vi "sensorsLoop.vi"() -> ()   [LabVIEW 2018]
uses:
  <vilib>/Rock Robotics/WPI/ThirdParty/Phoenix-LabVIEW/Motor Controller/Controls/CTRE_Phoenix_MotorControl_StatusFrameEnhanced.ctl
  <vilib>/Platform/TimedLoop/XDataNode/timing_clust.ctl
  <vilib>/Platform/TimedLoop/XDataNode/nitl_modes.ctl
  <vilib>/Platform/TimedLoop/XDataNode/wakeup.ctl
  Drive/driveShifterEnum.ctl
  Drive/MotionProfile/Constants.vi
  <vilib>/Rock Robotics/WPI/ThirdParty/Phoenix-LabVIEW/Motor Controller/Get/CTRE_Phoenix_MotorController_GetSelectedSensorData.vi
  <vilib>/Rock Robotics/WPI/ThirdParty/Phoenix-LabVIEW/Motor Controller/Get/CTRE_Phoenix_MotorController_GetQuadratureData.vi
  <vilib>/Rock Robotics/WPI/ThirdParty/Phoenix-LabVIEW/Pigeon IMU/CTRE_PigeonIMU_GetFusedHeading.vi
  <vilib>/Rock Robotics/WPI/ThirdParty/Phoenix-LabVIEW/Pigeon IMU/CTRE_PigeonIMU_GetBiasedAccelerometer.vi
  <vilib>/Rock Robotics/WPI/ThirdParty/Phoenix-LabVIEW/Pigeon IMU/CTRE_PigeonIMU_GetYPR.vi
  <vilib>/platform/TimedLoop/XDataNode/XDataNode.xnode
  <vilib>/Platform/TimedLoop/XDataNode/XDNodeRunTimeDep.lvlib
  <userlib>/836-Library/System/TDMS_V2/Support/TDMS_DevRef.ctl
  <userlib>/836-Library/System/TDMS_V2/Support/Logging_Settings.ctl
  <userlib>/836-Library/System/TDMS_V2/Support/Group_FIFO_Config.ctl
  <userlib>/836-Library/System/TDMS_V2/Support/Channel_FIFO_Config.ctl
panel:
  out "max 2":dbl
  out "velocity max_min 2":cluster{"min":dbl, "max":dbl, dbl}(graph)
  out "min 2":dbl
  out "Cal Status":T1
  in  "Read Enable":T2={"Cal Status"=TRUE, "Orientation"=TRUE, "Gyro"=FALSE, "Accelerometer"=FALSE, "Quanterion"=FALSE, "Accel Mode"=enum."Linear", "Magnetometer"=FALSE, "Register Mode"=enum."Quaternion"}
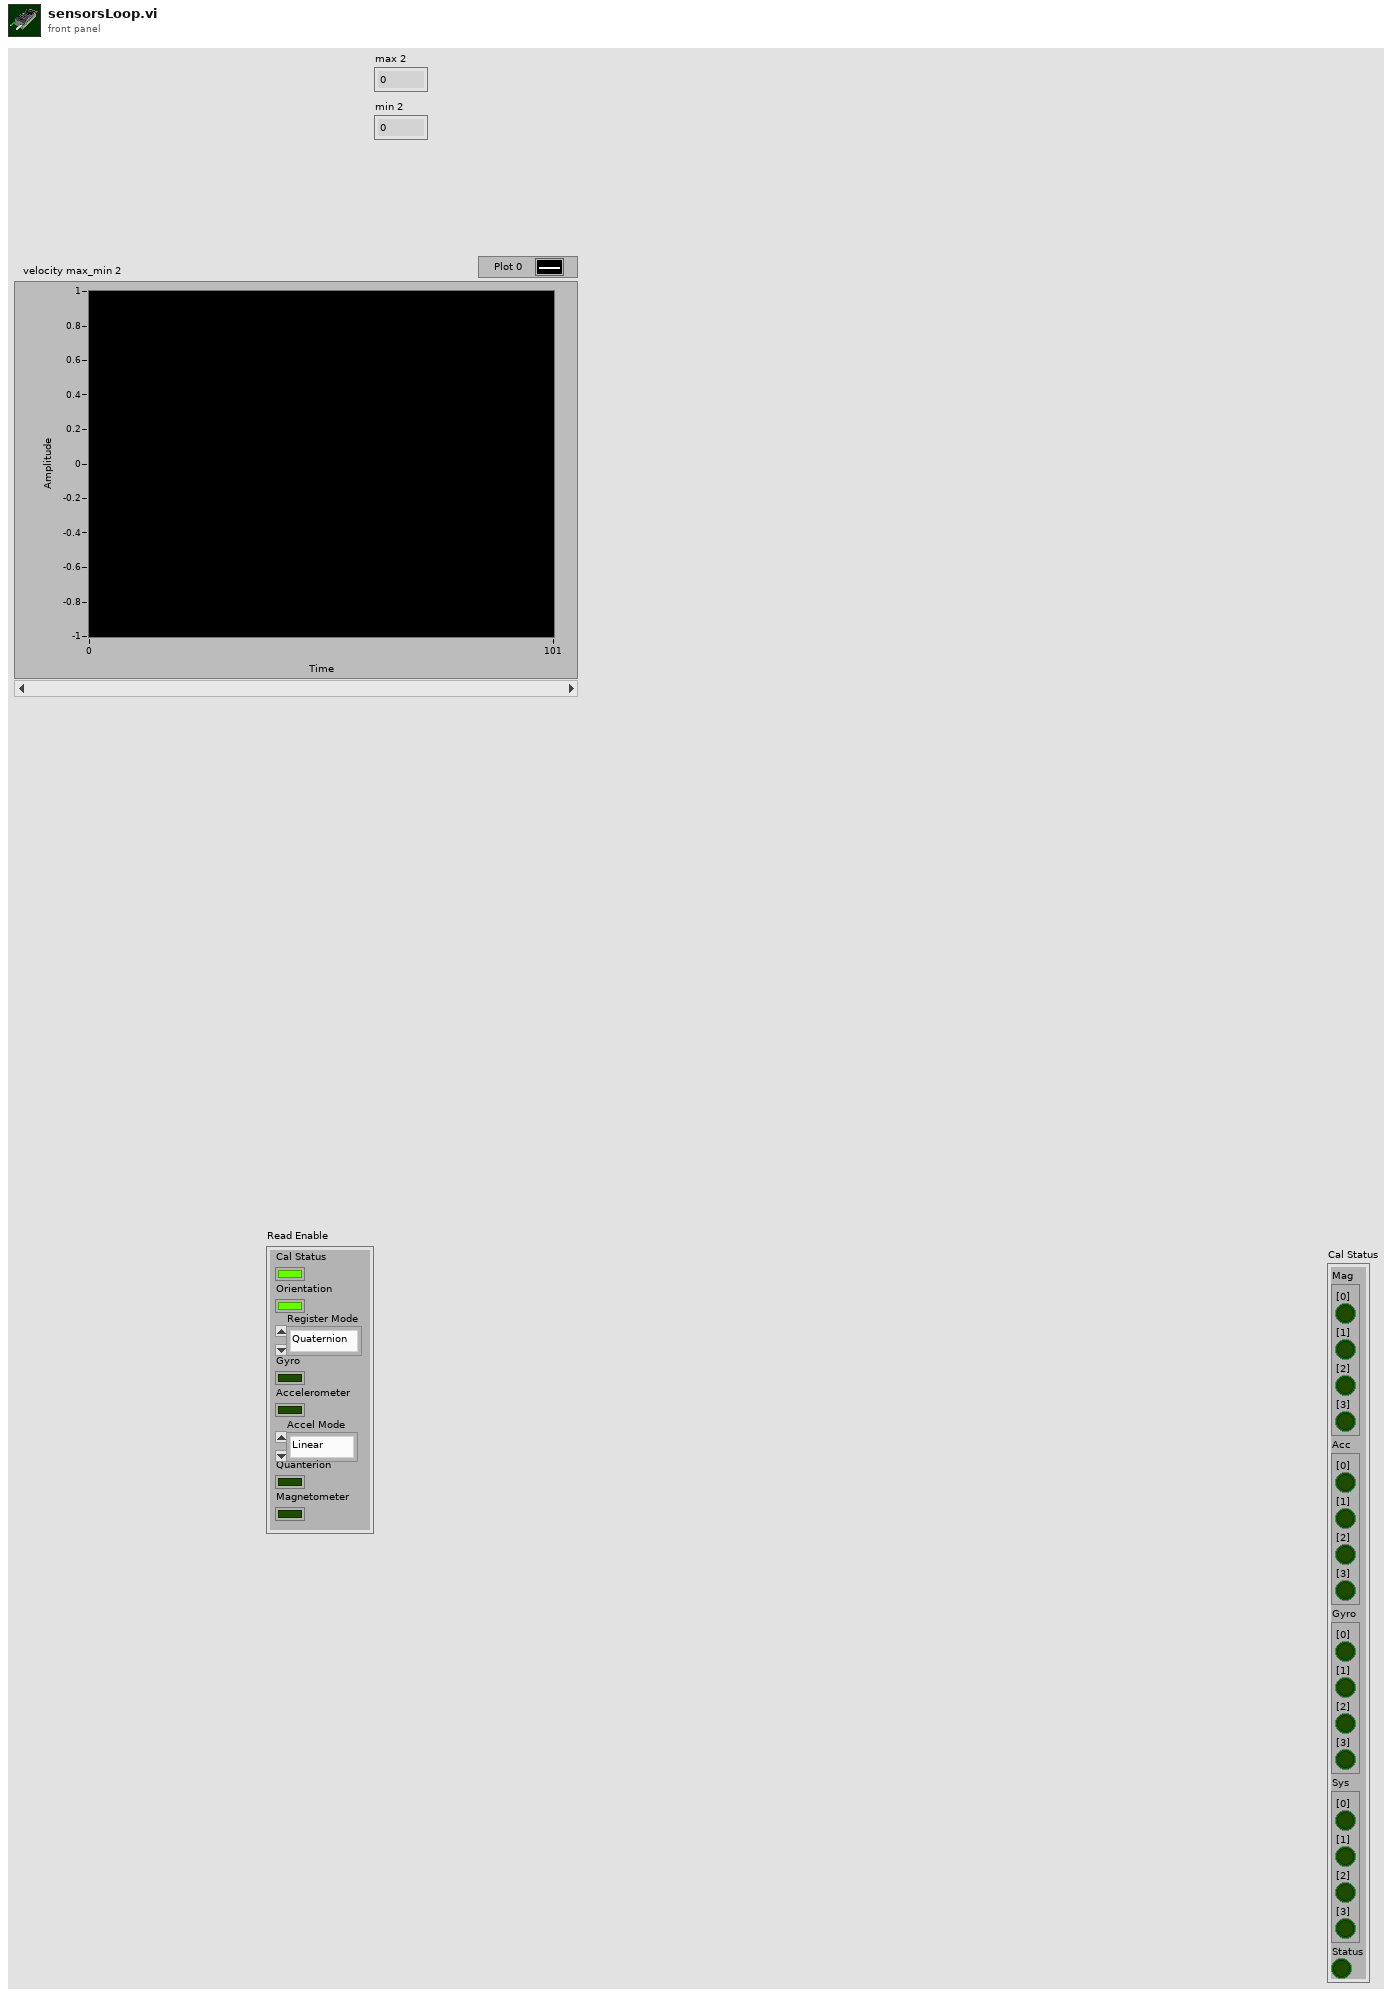
[diagram p1: front panel]
types:
  T1 = cluster{"Mag":cluster{"[0]":bool, "[1]":bool, "[2]":bool, "[3]":bool}, "Acc":cluster{"[0]":bool, "[1]":bool, "[2]":bool, "[3]":bool}, "Gyro":cluster{"[0]":bool, "[1]":bool, "[2]":bool, "[3]":bool}, "Sys":cluster{"[0]":bool, "[1]":bool, "[2]":bool, "[3]":bool}, "Status":bool}
  T2 = cluster{"Cal Status":bool, "Orientation":bool, "Gyro":bool, "Accelerometer":bool, "Quanterion":bool, "Accel Mode":enum8{"Raw Data", "Linear", "Gravity"}, "Magnetometer":bool, "Register Mode":enum8{"Euler", "Quaternion"}}
  T3 = typedef "CTRE_Phoenix_MotorControl_StatusFrameEnhanced.ctl" = u16
  T4 = typedef "WPI_MotorControlDeviceRef.ctl" = cluster{"DeviceStatus":errorcluster, "Type":T5, "PWM":cluster{"PWM Channel":T6, "DeadBand":T7}, "CAN":cluster{"Device Number":u8, "SetOutput VI Ref":variant, "GetOutput VI Ref":variant, "Enable VI Ref":variant, "Disable VI Ref":variant, "Data":variant}, "Invert":bool, "DIO PWM":cluster{"PWM \"Enable\" Channel":T6, "DIOChannel":T8, "PWM Rate":dbl}}
  T5 = typedef "WPI_MotorControlType.ctl" = enum16{"PWM", "CAN", "DIO PWM"}
  T6 = typedef "FPGA_DIOPWMChannel.ctl" = enum8{"PWM 0", "PWM 1", "PWM 2", "PWM 3", "PWM 4", "PWM 5", "PWM 6", "PWM 7", "PWM 8", "PWM 9", "PWM MXP 0", "PWM MXP 1", "PWM MXP 2", "PWM MXP 3", "PWM MXP 4", "PWM MXP 5", "PWM MXP 6", "PWM MXP 7", "PWM MXP 8", "PWM MXP 9", "Invalid"}
  T7 = typedef "WPI_PWMDeadband.ctl" = cluster{"Name":string, "maxPositivePwm":i32, "minPositivePwm":i32, "centerPwm":i32, "maxNegativePwm":i32, "minNegativePwm":i32, "angularRange":u16}
  T8 = typedef "FPGA_DIOChannel.ctl" = enum8{"DIO 0", "DIO 1", "DIO 2", "DIO 3", "DIO 4", "DIO 5", "DIO 6", "DIO 7", "DIO 8", "DIO 9", "DIO MXP 0", "DIO MXP 1", "DIO MXP 2", "DIO MXP 3", "DIO MXP 4", "DIO MXP 5", "DIO MXP 6", "DIO MXP 7", "DIO MXP 8", "DIO MXP 9", "DIO MXP 10", "DIO MXP 11", "DIO MXP 12", "DIO MXP 13", "DIO MXP 14", "DIO MXP 15", "SPI Port CS1", "SPI Port CS2", "SPI Port CS3", "SPI Port MISO", "SPI Port MOSI", "Invalid"}
  T9 = typedef "WPI_AnalogChannelDevRef.ctl" = cluster{"DevStatus":errorcluster, "Analog Channel":T10}
  T10 = typedef "FPGA_AIChannel.ctl" = enum8{"AI 0", "AI 1", "AI 2", "AI 3", "AI MXP 0", "AI MXP 1", "AI MXP 2", "AI MXP 3", "Invalid"}
  T11 = typedef "CTRE_PigeonIMU_DeviceRef.ctl" = cluster{"DeviceStatus":errorcluster, "Device Number":u8, "Type":T12, "Device ID":u32, "Handle":u64, "UsageFrame":u32, "Library Path":path}
  T12 = typedef "CTRE_PigeonIMU_ConnectionType.ctl" = u32
  T13 = typedef "WPI_DigitalInputDevRef.ctl" = cluster{"DevStatus":errorcluster, "DIO Channel":T8}
  T14 = typedef "XDNodeRunTimeDep.lvlib/timing_clust.ctl" = cluster{"Expected End [f-1]":u64, "Actual End [f-1]":u64, "Finished Late? [f-1]":bool, "Expected End [i-1]":u64, "Actual End [i-1]":u64, "Finished Late? [i-1]":bool, "Expected Start [i]":u64, "Actual Start [i]":u64, "Expected Start [f]":u64, "Actual Start [f]":u64, "Source Name":string, "Structure Name":string, "Period":i64, "Deadline":i64, "Offset":i64, "Start":i64, "Priority":i32, "Timeout":i32, "Mode":T15, "Wakeup Reason":T16, "Error":errorcluster, "Source Type":string, "Secondary Source Type":string, "Global End Time":u64, "Global Start Time":u64, "Frame Duration":u64, "Iteration Duration":u64, "Assigned CPU":i32, "I/O Scan Engine Mode":u32}
  T15 = typedef "XDNodeRunTimeDep.lvlib/nitl_modes.ctl" = enum32{"No Change", "Process missed periods, maintain original phase", "Discard missed periods, maintain original phase", "Process missed periods, ignore original phase", "Discard missed periods, ignore original phase"}
  T16 = typedef "XDNodeRunTimeDep.lvlib/wakeup.ctl" = enum32{"Normal", "Aborted", "Asynchronous wakeup", "Timing source error", "Timed loop error", "Timeout"}
  T17 = typedef "ImuDevRef.ctl" = cluster{"I2CDevRef":T18, "Valid Cal File?":bool}
  T18 = typedef "WPI_I2CDevRef.ctl" = cluster{"DevStatus":errorcluster, "Device Address":u8, "Handle":i32, "I2C Bus":T19}
  T19 = typedef "i2c_bus.ctl" = enum16{"I2C On-Board", "I2C MXP", "Invalid"}
  T20 = enum16{"Inches -> Sensor Units", "Sensor Units -> Inches"}
  T21 = typedef "driveShifterEnum.ctl" = enum16{"Low", "High"}
  T22 = cluster{"Heading":dbl, "Valid?":bool, "Fusing?":bool}
  T23 = typedef "TDMS_DevRef.ctl" = cluster{"Name":string, "File Ref":refnum<k34>, "Start Time":timestamp, "Logging Settings":T24, "Group FIFO Config":T25[], "Data To Write":refnum<data-value>, "semaphore":T27, "Ref Time Reset":refnum<k4>}
  T24 = typedef "Logging_Settings.ctl" = cluster{"Data Grab Period":dbl, "File Write Period":dbl, "Max Stored Size":dbl, "Burst Size":dbl}
  T25 = typedef "Group_FIFO_Config.ctl" = cluster{"Group":string, "Channels":T26[], "Channel Names":string[]}
  T26 = typedef "Channel_FIFO_Config.ctl" = cluster{"Channel":string, "FIFO":refnum<k33>}
  T27 = typedef "Semaphore RefNum" = refnum<k1>
  T28 = cluster{"Yaw":dbl, "Roll":dbl, "Pitch":dbl, "Yaw Wind":dbl, "Roll Wind":dbl, "Pitch Wind":dbl}
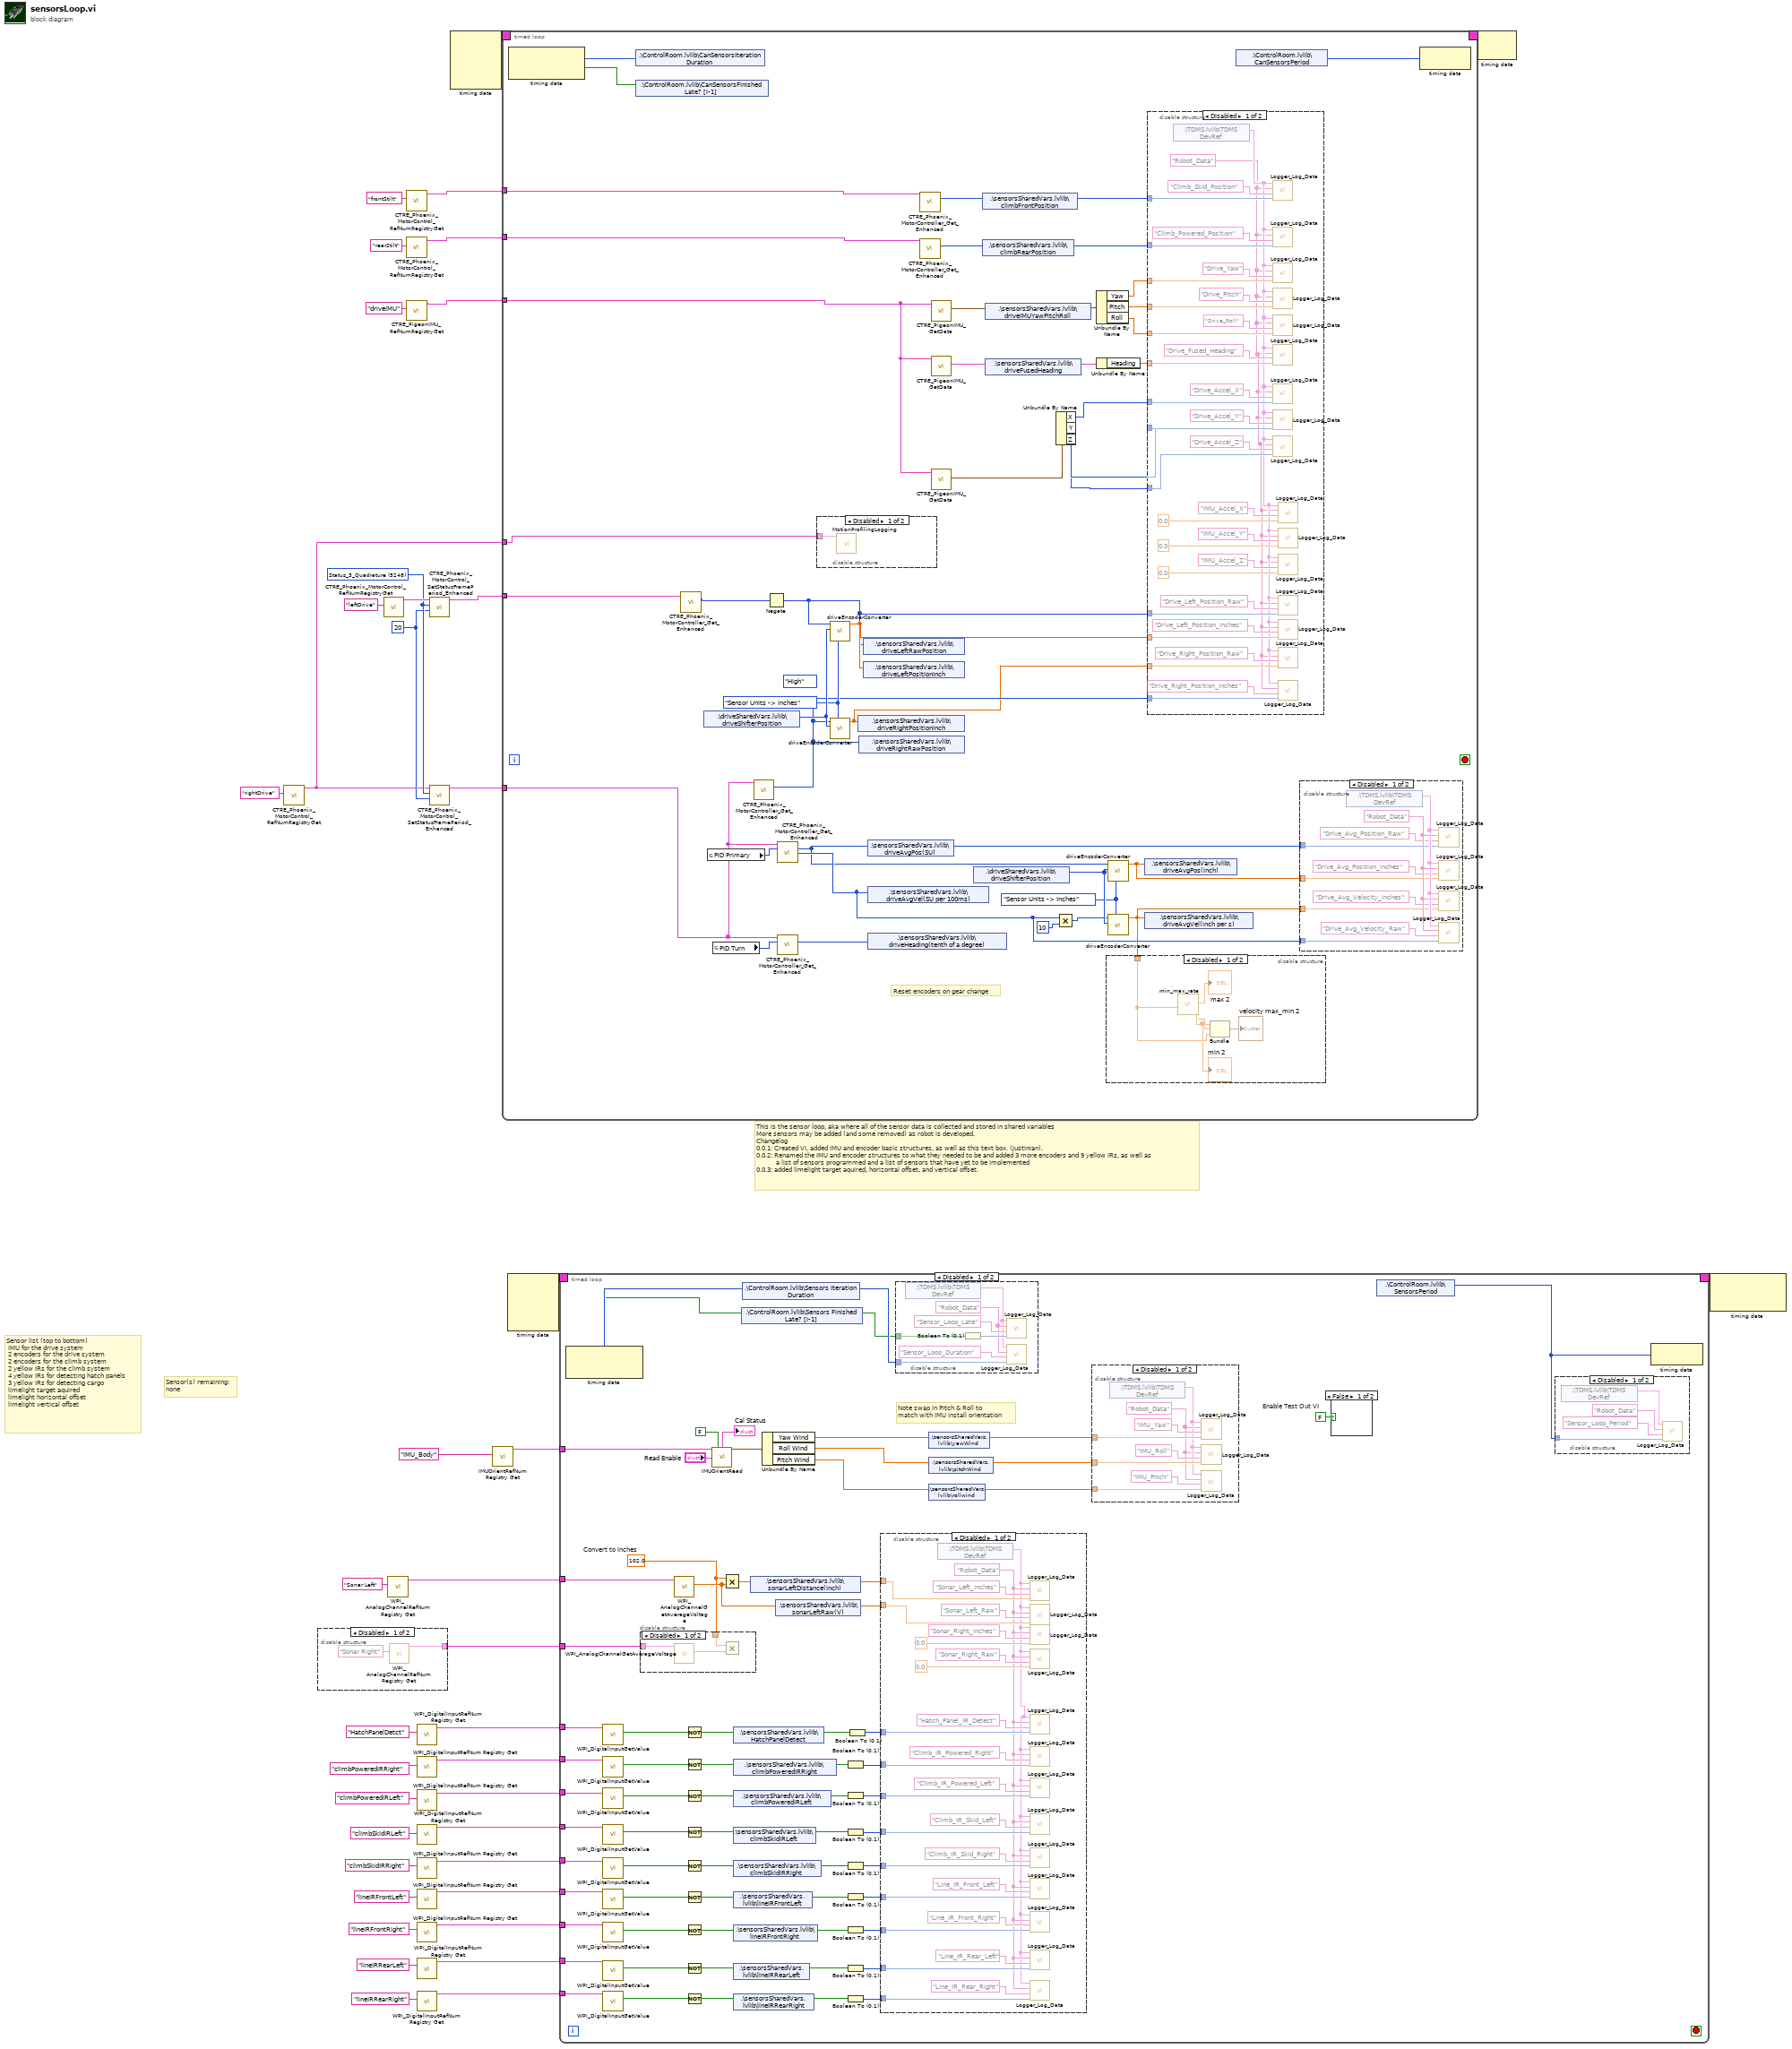
[diagram p0: block diagram]
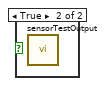
[diagram p12: hidden frame]
diagram:
  w4 = 20 ("periodMs")
  w5 = T3 5248 items=["Status_1_General"=5120, "Status_2_Feedback0"=5184, "Status_3_Quadrature"=5248, "Status_4_AinTempVbat"=5312, "Status_6_Misc"=5440, "Status_7_CommStatus"=5504, "Status_8_PulseWidth"=5568, "Status_9_MotProfBuffer"=5632, "Status_10_MotionMagic"=5696, "Status_11_UartGadgeteer"=5760, "Status_12_Feedback1"=5824, "Status_13_Base_PIDF0"=5888, "Status_14_Turn_PIDF1"=5952, "Status_15_FirmwareApiStatus"=6016] ("Status Frame")
  # "Sensor(s) remaining:\nnone"
  # "Sensor list (top to bottom)\n IMU for the drive system\n 2 encoders for the drive system\n 2 encoders for the climb system\n 2 yellow IRs for the climb system\n 4 yellow IRs for detecting hatch panels\n 3 yellow IRs for detecting cargo\n limelight target aquired\n limelight horizontal offset\n limelight vertical offset"
  # "This is the sensor loop, aka where all of the sensor data is collected and stored in shared variables\nMore sensors may be added (and some removed) as robot is developed.\nChangelog\n0.0.1: Created VI, added IMU and encoder basic structures, as well as this text box. (Justinian).\n0.0.2: Renamed the IMU and encoder structures to what they needed to be and added 3 more encoders and 9 yellow IRs, as well as\n           a list of sensors programmed and a list of sensors that have yet to be implemented\n0.0.3: added limelight target aquired, horizontal offset, and vertical offset."
  n1 = call <vilib>:"CTRE_Phoenix_MotorControl_RefNumRegistryGet.vi"("refnum name"="rightDrive") -> ("PhoenixMotorControlDevRef"=w2:T4)  [unwired: 9 in, 1 out]
  n2 = disable-structure shown="Disabled" {
    disable-tunnel: [w43 _] -> w19
    frame Disabled {
      n3 = call <vilib>:"WPI_AnalogChannelRefNum Registry Get.vi"("refnum name"="Sonar Right") -> ("AIDeviceRef"=w43:T9)  [unwired: 9 in, 1 out]
    }
    frame Enabled {
    }
  }
  n4 = call <vilib>:"CTRE_Phoenix_MotorControl_RefNumRegistryGet.vi"("refnum name"="leftDrive") -> ("PhoenixMotorControlDevRef"=w6:T4)  [unwired: 9 in, 1 out]
  n5 = call <vilib>:"WPI_AnalogChannelRefNum Registry Get.vi"("refnum name"="Sonar Left") -> ("AIDeviceRef"=w20:T9)  [unwired: 9 in, 1 out]
  n6 = call <vilib>:"CTRE_Phoenix_MotorControl_RefNumRegistryGet.vi"("refnum name"="frontStilt") -> ("PhoenixMotorControlDevRef"=w11:T4)  [unwired: 9 in, 1 out]
  n7 = call <vilib>:"CTRE_Phoenix_MotorControl_RefNumRegistryGet.vi"("refnum name"="rearStilt") -> ("PhoenixMotorControlDevRef"=w10:T4)  [unwired: 9 in, 1 out]
  n8 = call <vilib>:"CTRE_PigeonIMU_RefNumRegistryGet.vi"("refnum name"="driveIMU") -> ("PigeonIMUDevRef"=w9:T11)  [unwired: 9 in, 1 out]
  n9 = call <vilib>:"WPI_DigitalInputRefNum Registry Get.vi"("refnum name"="HatchPanelDetct") -> ("DigitalInputDevRef"=w17:T13)  [unwired: 9 in, 1 out]
  n10 = call <vilib>:"WPI_DigitalInputRefNum Registry Get.vi"("refnum name"="climbPoweredIRRight") -> ("DigitalInputDevRef"=w30:T13)  [unwired: 9 in, 1 out]
  n11 = call <vilib>:"WPI_DigitalInputRefNum Registry Get.vi"("refnum name"="climbPoweredIRLeft") -> ("DigitalInputDevRef"=w29:T13)  [unwired: 9 in, 1 out]
  n12 = call <vilib>:"WPI_DigitalInputRefNum Registry Get.vi"("refnum name"="climbSkidIRLeft") -> ("DigitalInputDevRef"=w28:T13)  [unwired: 9 in, 1 out]
  n13 = call <vilib>:"WPI_DigitalInputRefNum Registry Get.vi"("refnum name"="climbSkidIRRight") -> ("DigitalInputDevRef"=w27:T13)  [unwired: 9 in, 1 out]
  n14 = call <vilib>:"WPI_DigitalInputRefNum Registry Get.vi"("refnum name"="lineIRFrontLeft") -> ("DigitalInputDevRef"=w26:T13)  [unwired: 9 in, 1 out]
  n15 = call <vilib>:"WPI_DigitalInputRefNum Registry Get.vi"("refnum name"="lineIRFrontRight") -> ("DigitalInputDevRef"=w25:T13)  [unwired: 9 in, 1 out]
  n16 = call <vilib>:"WPI_DigitalInputRefNum Registry Get.vi"("refnum name"="lineIRRearLeft") -> ("DigitalInputDevRef"=w24:T13)  [unwired: 9 in, 1 out]
  n17 = call <vilib>:"WPI_DigitalInputRefNum Registry Get.vi"("refnum name"="lineIRRearRight") -> ("DigitalInputDevRef"=w23:T13)  [unwired: 9 in, 1 out]
  n18 = call <vilib>:"CTRE_Phoenix_MotorControl_SetStatusFramePeriod_Enhanced.vi"("periodMs"=w4, "Status Frame"=w5, "PhoenixMotorControlDevRef"=w6) -> ("PhoenixMotorControlDevRef"=w3:T4)  [unwired: 7 in, 1 out]
  n19 = call <vilib>:"CTRE_Phoenix_MotorControl_SetStatusFramePeriod_Enhanced.vi"("periodMs"=w4, "Status Frame"=w5, "PhoenixMotorControlDevRef"=w2) -> ("PhoenixMotorControlDevRef"=w1:T4)  [unwired: 7 in, 1 out]
  n20 = node-c288() -> (w16:T14)  [unwired: 4 in]
  n21 = call <userlib>:"IMUOrientRefNum Registry Get.vi"("refnum name"="IMU_Body") -> ("IMUDevRef out"=w39:T17)  [unwired: 9 in, 1 out]
  n22 = timed-loop {
    timing: w16 -> [_]
    timing-out: [_] -> w15
    tunnel: w11 -> [w70]
    tunnel: w10 -> [w69]
    tunnel: w9 -> [w68]
    tunnel: w3 -> [w54]
    tunnel: w2 -> [w56]
    tunnel: w1 -> [w55]
    stop <- _ stop-if-true
    w47 = T20."Sensor Units -> Inches" ("Conversion Direction")
    (unwired) enum16{"High", "Low"}."High" ("Gear Setting")
    w66 = T20."Sensor Units -> Inches" ("Conversion Direction")
    # "Reset encoders on gear change"
    n23 = node-c288() -> (w53:i64, w52:bool)  [unwired: 1 in]
    n24 = shared-variable ".\\ControlRoom.lvlib\\CanSensorsIteration Duration"(w53) -> ()  [unwired: 1 in, 1 out]
    n25 = shared-variable ".\\ControlRoom.lvlib\\CanSensorsFinished Late? [i-1]"(w52) -> ()  [unwired: 1 in, 1 out]
    n26 = call-poly <vilib>:"CTRE_Phoenix_MotorController_Get_Enhanced.vi"("PhoenixMotorControlDevRef"=w54) -> ("Quadrature Position"=w58:i32)  [unwired: 11 in, 3 out]
    n27 = shared-variable ".\\driveSharedVars.lvlib\\driveShifterPosition"() -> (w67:T21)  [unwired: 1 in, 1 out]
    n28 = global read "Constants.vi" "PID Primary"() -> (w44:i32)
    n29 = global read "Constants.vi" "PID Turn"() -> (w45:i32)
    n30 = call-poly <vilib>:"CTRE_Phoenix_MotorController_Get_Enhanced.vi"("PhoenixMotorControlDevRef"=w55) -> ("Quadrature Position"=w62:i32)  [unwired: 11 in, 3 out]
    n31 = Negate(x=w58) -> (-x=w59:i32)
    n32 = call-poly <vilib>:"CTRE_Phoenix_MotorController_Get_Enhanced.vi"("PhoenixMotorControlDevRef"=w55, "pidLoopIdx"=w44) -> ("Position (Raw Sensor Units)"=w63:i32, "Velocity (Raw Sensor Units per 100 ms)"=w65:i32)  [unwired: 10 in, 2 out]
    n33 = call-poly <vilib>:"CTRE_Phoenix_MotorController_Get_Enhanced.vi"("PhoenixMotorControlDevRef"=w55, "pidLoopIdx"=w45) -> ("Position (Raw Sensor Units)"=w46:i32)  [unwired: 10 in, 3 out]
    n34 = disable-structure shown="Disabled" {
      disable-tunnel: w56 -> [w127 _]
      frame Disabled {
        n35 = call "MotionProfilingLogging.vi"("Main Talon"=w127) -> ()  [unwired: 11 in]
      }
      frame Enabled {
      }
    }
    n36 = call "driveEncoderConverter.vi"("Conversion Direction"=w66, "Gear Setting"=w67, "Input"=w59) -> ("Output"=w60:dbl)  [unwired: 8 in]
    n37 = call "driveEncoderConverter.vi"("Conversion Direction"=w66, "Gear Setting"=w67, "Input"=w62) -> ("Output"=w61:dbl)  [unwired: 8 in]
    n38 = shared-variable ".\\sensorsSharedVars.lvlib\\driveRightPositionInch"(w61) -> ()  [unwired: 1 in, 1 out]
    n39 = shared-variable ".\\sensorsSharedVars.lvlib\\driveRightRawPosition"(w62) -> ()  [unwired: 1 in, 1 out]
    n40 = shared-variable ".\\sensorsSharedVars.lvlib\\driveLeftPositionInch"(w60) -> ()  [unwired: 1 in, 1 out]
    n41 = shared-variable ".\\sensorsSharedVars.lvlib\\driveLeftRawPosition"(w59) -> ()  [unwired: 1 in, 1 out]
    n42 = shared-variable ".\\sensorsSharedVars.lvlib\\driveAvgPos(SU)"(w63) -> ()  [unwired: 1 in, 1 out]
    n43 = shared-variable ".\\sensorsSharedVars.lvlib\\driveAvgVel(SU per 100ms)"(w65) -> ()  [unwired: 1 in, 1 out]
    n44 = shared-variable ".\\sensorsSharedVars.lvlib\\driveHeading(tenth of a degree)"(w46) -> ()  [unwired: 1 in, 1 out]
    n45 = call-poly <vilib>:"CTRE_Phoenix_MotorController_Get_Enhanced.vi"("PhoenixMotorControlDevRef"=w70) -> ("Position (Raw Sensor Units)"=w82:i32)  [unwired: 11 in, 3 out]
    n46 = call-poly <vilib>:"CTRE_Phoenix_MotorController_Get_Enhanced.vi"("PhoenixMotorControlDevRef"=w69) -> ("Position (Raw Sensor Units)"=w81:i32)  [unwired: 11 in, 3 out]
    n47 = call-poly <vilib>:"CTRE_PigeonIMU_GetData.vi"("PigeonIMUDevRef"=w68) -> ("Yaw Pitch Roll"=w72:cluster{"Yaw":dbl, "Pitch":dbl, "Roll":dbl})  [unwired: 8 in, 2 out]
    n48 = call-poly <vilib>:"CTRE_PigeonIMU_GetData.vi"("PigeonIMUDevRef"=w68) -> ("Fused Heading"=w71:T22)  [unwired: 8 in, 2 out]
    n49 = call-poly <vilib>:"CTRE_PigeonIMU_GetData.vi"("PigeonIMUDevRef"=w68) -> ("Biased Accelerometer"=w76:cluster{"X":i16, "Y":i16, "Z":i16, "Norm":i16})  [unwired: 8 in, 2 out]
    n50 = shared-variable ".\\driveSharedVars.lvlib\\driveShifterPosition"() -> (w50:T21)  [unwired: 1 in, 1 out]
    n51 = shared-variable ".\\sensorsSharedVars.lvlib\\climbFrontPosition"(w82) -> ()  [unwired: 1 in, 1 out]
    n52 = shared-variable ".\\sensorsSharedVars.lvlib\\climbRearPosition"(w81) -> ()  [unwired: 1 in, 1 out]
    n53 = shared-variable ".\\sensorsSharedVars.lvlib\\driveIMUYawPitchRoll"(w72) -> ()  [unwired: 1 in, 1 out]
    n54 = shared-variable ".\\sensorsSharedVars.lvlib\\driveFusedHeading"(w71) -> ()  [unwired: 1 in, 1 out]
    n55 = Multiply(x=w65, y=10) -> (x*y=w48:i32)
    n56 = Unbundle By Name(w76) -> ("X"=w74:i16, "Y"=w75:i16, "Z"=w73:i16)
    n57 = Unbundle By Name(w72) -> ("Yaw"=w80:dbl, "Pitch"=w79:dbl, "Roll"=w78:dbl)
    n58 = Unbundle By Name(w71) -> ("Heading"=w77:dbl)
    n59 = call "driveEncoderConverter.vi"("Conversion Direction"=w47, "Gear Setting"=w50, "Input"=w63) -> ("Output"=w64:dbl)  [unwired: 8 in]
    n60 = call "driveEncoderConverter.vi"("Conversion Direction"=w47, "Gear Setting"=w50, "Input"=w48) -> ("Output"=w57:dbl)  [unwired: 8 in]
    n61 = disable-structure shown="Disabled" {
      disable-tunnel: w57 -> [w131 _]
      frame Disabled {
        n62 = call "min_max_rate.vi"("Rate"=w131) -> ("min"=w130:dbl, "max"=w129:dbl)  [unwired: 9 in]
        "min 2" <- w130
        "max 2" <- w129
        n63 = Bundle("min"=w130, "max"=w129, "Output"=w131) -> (→"velocity max_min 2":cluster{"min":dbl, "max":dbl, "Output":dbl})  [unwired: 1 in]
      }
      frame Enabled {
      }
    }
    n64 = shared-variable ".\\sensorsSharedVars.lvlib\\driveAvgPos(inch)"(w64) -> ()  [unwired: 1 in, 1 out]
    n65 = shared-variable ".\\sensorsSharedVars.lvlib\\driveAvgVel(inch per s)"(w57) -> ()  [unwired: 1 in, 1 out]
    n66 = disable-structure shown="Disabled" {
      disable-tunnel: w82 -> [w126 _]
      disable-tunnel: w81 -> [w125 _]
      disable-tunnel: w80 -> [w124 _]
      disable-tunnel: w79 -> [w123 _]
      disable-tunnel: w78 -> [w122 _]
      disable-tunnel: w77 -> [w121 _]
      disable-tunnel: w75 -> [w120 _]
      disable-tunnel: w74 -> [w119 _]
      disable-tunnel: w73 -> [w118 _]
      disable-tunnel: w62 -> [w98 _]
      disable-tunnel: w61 -> [w97 _]
      disable-tunnel: w60 -> [w96 _]
      disable-tunnel: w59 -> [w95 _]
      frame Disabled {
        w93 = "Robot_Data" ("Group")
        n67 = shared-variable ".\\TDMS.lvlib\\TDMS DevRef"() -> (w94:T23)  [unwired: 1 in, 1 out]
        n68 = call <userlib>:"Logger_Log_Data.vi"("Data"=w126, "Channel"="Climb_Skid_Position", "Group"=w93, "TDMS DevRef"=w94) -> ()  [unwired: 7 in, 1 out]
        n69 = call <userlib>:"Logger_Log_Data.vi"("Data"=w125, "Channel"="Climb_Powered_Position", "Group"=w93, "TDMS DevRef"=w94) -> ()  [unwired: 7 in, 1 out]
        n70 = call <userlib>:"Logger_Log_Data.vi"("Data"=w124, "Channel"="Drive_Yaw", "Group"=w93, "TDMS DevRef"=w94) -> ()  [unwired: 7 in, 1 out]
        n71 = call <userlib>:"Logger_Log_Data.vi"("Data"=w123, "Channel"="Drive_Pitch", "Group"=w93, "TDMS DevRef"=w94) -> ()  [unwired: 7 in, 1 out]
        n72 = call <userlib>:"Logger_Log_Data.vi"("Data"=w122, "Channel"="Drive_Roll", "Group"=w93, "TDMS DevRef"=w94) -> ()  [unwired: 7 in, 1 out]
        n73 = call <userlib>:"Logger_Log_Data.vi"("Data"=w121, "Channel"="Drive_Fused_Heading", "Group"=w93, "TDMS DevRef"=w94) -> ()  [unwired: 7 in, 1 out]
        n74 = call <userlib>:"Logger_Log_Data.vi"("Data"=w119, "Channel"="Drive_Accel_X", "Group"=w93, "TDMS DevRef"=w94) -> ()  [unwired: 7 in, 1 out]
        n75 = call <userlib>:"Logger_Log_Data.vi"("Data"=w120, "Channel"="Drive_Accel_Y", "Group"=w93, "TDMS DevRef"=w94) -> ()  [unwired: 7 in, 1 out]
        n76 = call <userlib>:"Logger_Log_Data.vi"("Data"=w118, "Channel"="Drive_Accel_Z", "Group"=w93, "TDMS DevRef"=w94) -> ()  [unwired: 7 in, 1 out]
        n77 = call <userlib>:"Logger_Log_Data.vi"("Data"=0.0, "Channel"="IMU_Accel_X", "Group"=w93, "TDMS DevRef"=w94) -> ()  [unwired: 7 in, 1 out]
        n78 = call <userlib>:"Logger_Log_Data.vi"("Data"=0.0, "Channel"="IMU_Accel_Y", "Group"=w93, "TDMS DevRef"=w94) -> ()  [unwired: 7 in, 1 out]
        n79 = call <userlib>:"Logger_Log_Data.vi"("Data"=0.0, "Channel"="IMU_Accel_Z", "Group"=w93, "TDMS DevRef"=w94) -> ()  [unwired: 7 in, 1 out]
        n80 = call <userlib>:"Logger_Log_Data.vi"("Data"=w95, "Channel"="Drive_Left_Position_Raw", "Group"=w93, "TDMS DevRef"=w94) -> ()  [unwired: 7 in, 1 out]
        n81 = call <userlib>:"Logger_Log_Data.vi"("Data"=w96, "Channel"="Drive_Left_Position_Inches", "Group"=w93, "TDMS DevRef"=w94) -> ()  [unwired: 7 in, 1 out]
        n82 = call <userlib>:"Logger_Log_Data.vi"("Data"=w97, "Channel"="Drive_Right_Position_Raw", "Group"=w93, "TDMS DevRef"=w94) -> ()  [unwired: 7 in, 1 out]
        n83 = call <userlib>:"Logger_Log_Data.vi"("Data"=w98, "Channel"="Drive_Right_Position_Inches", "Group"=w93, "TDMS DevRef"=w94) -> ()  [unwired: 7 in, 1 out]
      }
      frame Enabled {
      }
    }
    n84 = shared-variable ".\\ControlRoom.lvlib\\CanSensorsPeriod"() -> (w51:i64)  [unwired: 1 in, 1 out]
    n85 = disable-structure shown="Disabled" {
      disable-tunnel: w65 -> [w86 _]
      disable-tunnel: w64 -> [w85 _]
      disable-tunnel: w63 -> [w84 _]
      disable-tunnel: w57 -> [w83 _]
      frame Disabled {
        w92 = "Robot_Data" ("Group")
        n86 = shared-variable ".\\TDMS.lvlib\\TDMS DevRef"() -> (w91:T23)  [unwired: 1 in, 1 out]
        n87 = call <userlib>:"Logger_Log_Data.vi"("Data"=w84, "Channel"="Drive_Avg_Position_Raw", "Group"=w92, "TDMS DevRef"=w91) -> ()  [unwired: 7 in, 1 out]
        n88 = call <userlib>:"Logger_Log_Data.vi"("Data"=w85, "Channel"="Drive_Avg_Position_Inches", "Group"=w92, "TDMS DevRef"=w91) -> ()  [unwired: 7 in, 1 out]
        n89 = call <userlib>:"Logger_Log_Data.vi"("Data"=w83, "Channel"="Drive_Avg_Velocity_Inches", "Group"=w92, "TDMS DevRef"=w91) -> ()  [unwired: 7 in, 1 out]
        n90 = call <userlib>:"Logger_Log_Data.vi"("Data"=w86, "Channel"="Drive_Avg_Velocity_Raw", "Group"=w92, "TDMS DevRef"=w91) -> ()  [unwired: 7 in, 1 out]
      }
      frame Enabled {
      }
    }
    n91 = node-c288(w51) -> ()  [unwired: 1 out]
  }
  n92 = node-c288() -> (w41:T14)  [unwired: 4 in]
  n93 = timed-loop {
    timing: w41 -> [_]
    timing-out: [_] -> w40
    tunnel: w39 -> [w182]
    tunnel: w30 -> [w190]
    tunnel: w29 -> [w189]
    tunnel: w28 -> [w188]
    tunnel: w27 -> [w187]
    tunnel: w26 -> [w186]
    tunnel: w25 -> [w185]
    tunnel: w24 -> [w184]
    tunnel: w23 -> [w183]
    tunnel: w20 -> [w181]
    tunnel: w19 -> [w180]
    tunnel: w17 -> [w179]
    stop <- _ stop-if-true
    w138 = 102.0  # Convert to Inches
    w175 = FALSE  # Enable Test Out VI
    # "Note swap in Pitch & Roll to\nmatch with IMU install orientation"
    n94 = node-c288() -> (w177:i64, w176:bool)  [unwired: 1 in]
    n95 = call <vilib>:"WPI_DigitalInputGetValue.vi"("DigitalInputDevRef"=w179) -> ("Value"=w159:bool)  [unwired: 8 in, 2 out]
    n96 = call <vilib>:"WPI_DigitalInputGetValue.vi"("DigitalInputDevRef"=w190) -> ("Value"=w167:bool)  [unwired: 8 in, 2 out]
    n97 = call <vilib>:"WPI_DigitalInputGetValue.vi"("DigitalInputDevRef"=w189) -> ("Value"=w166:bool)  [unwired: 8 in, 2 out]
    n98 = call <vilib>:"WPI_DigitalInputGetValue.vi"("DigitalInputDevRef"=w188) -> ("Value"=w165:bool)  [unwired: 8 in, 2 out]
    n99 = call <vilib>:"WPI_DigitalInputGetValue.vi"("DigitalInputDevRef"=w187) -> ("Value"=w164:bool)  [unwired: 8 in, 2 out]
    n100 = call <vilib>:"WPI_DigitalInputGetValue.vi"("DigitalInputDevRef"=w186) -> ("Value"=w163:bool)  [unwired: 8 in, 2 out]
    n101 = call <vilib>:"WPI_DigitalInputGetValue.vi"("DigitalInputDevRef"=w185) -> ("Value"=w162:bool)  [unwired: 8 in, 2 out]
    n102 = call <vilib>:"WPI_DigitalInputGetValue.vi"("DigitalInputDevRef"=w184) -> ("Value"=w161:bool)  [unwired: 8 in, 2 out]
    n103 = call <vilib>:"WPI_DigitalInputGetValue.vi"("DigitalInputDevRef"=w183) -> ("Value"=w160:bool)  [unwired: 8 in, 2 out]
    n104 = disable-structure shown="Disabled" {
      disable-tunnel: w180 -> [w240 _]
      disable-tunnel: w138 -> [w239 _]
      frame Disabled {
        n105 = call <vilib>:"WPI_AnalogChannelGetAverageVoltage.vi"("AIDeviceRef"=w240) -> ("Voltage"=w238:dbl)  [unwired: 8 in, 2 out]
        n106 = Multiply(x=w239, y=w238) -> ()  [unwired: 1 out]
      }
      frame Enabled {
      }
    }
    n107 = call <vilib>:"WPI_AnalogChannelGetAverageVoltage.vi"("AIDeviceRef"=w181) -> ("Voltage"=w157:dbl)  [unwired: 8 in, 2 out]
    n108 = Not(x=w159) -> (.not. x?=w156:bool)
    n109 = Not(x=w167) -> (.not. x?=w155:bool)
    n110 = Not(x=w166) -> (.not. x?=w154:bool)
    n111 = Not(x=w165) -> (.not. x?=w153:bool)
    n112 = Not(x=w164) -> (.not. x?=w152:bool)
    n113 = Not(x=w163) -> (.not. x?=w151:bool)
    n114 = Not(x=w162) -> (.not. x?=w150:bool)
    n115 = Not(x=w161) -> (.not. x?=w149:bool)
    n116 = Not(x=w160) -> (.not. x?=w148:bool)
    n117 = call <userlib>:"IMUOrientRead.vi"("IMU Dev Ref"=w182, "Orient Reset (Wind)"=FALSE, "Read Enable"="Read Enable") -> ("Cal Status"=→"Cal Status":T1, "Orient Y/R/P"=w171:T28)  [unwired: 5 in, 6 out]
    n118 = Multiply(x=w138, y=w157) -> (x*y=w158:dbl)
    n119 = shared-variable ".\\sensorsSharedVars.lvlib\\HatchPanelDetect"(w156) -> ()  [unwired: 1 in, 1 out]
    n120 = shared-variable ".\\sensorsSharedVars.lvlib\\climbPoweredIRRight"(w155) -> ()  [unwired: 1 in, 1 out]
    n121 = shared-variable ".\\sensorsSharedVars.lvlib\\climbPoweredIRLeft"(w154) -> ()  [unwired: 1 in, 1 out]
    n122 = shared-variable ".\\sensorsSharedVars.lvlib\\climbSkidIRLeft"(w153) -> ()  [unwired: 1 in, 1 out]
    n123 = shared-variable ".\\sensorsSharedVars.lvlib\\climbSkidIRRight"(w152) -> ()  [unwired: 1 in, 1 out]
    n124 = shared-variable ".\\sensorsSharedVars.lvlib\\lineIRFrontLeft"(w151) -> ()  [unwired: 1 in, 1 out]
    n125 = shared-variable ".\\sensorsSharedVars.lvlib\\lineIRFrontRight"(w150) -> ()  [unwired: 1 in, 1 out]
    n126 = shared-variable ".\\sensorsSharedVars.lvlib\\lineIRRearLeft"(w149) -> ()  [unwired: 1 in, 1 out]
    n127 = shared-variable ".\\sensorsSharedVars.lvlib\\lineIRRearRight"(w148) -> ()  [unwired: 1 in, 1 out]
    n128 = shared-variable ".\\ControlRoom.lvlib\\Sensors Finished Late? [i-1]"(w176) -> ()  [unwired: 1 in, 1 out]
    n129 = shared-variable ".\\ControlRoom.lvlib\\Sensors Iteration Duration"(w177) -> ()  [unwired: 1 in, 1 out]
    n130 = shared-variable ".\\sensorsSharedVars.lvlib\\sonarLeftDistance(inch)"(w158) -> ()  [unwired: 1 in, 1 out]
    n131 = Unbundle By Name(w171) -> ("Yaw Wind"=w174:dbl, "Roll Wind"=w173:dbl, "Pitch Wind"=w172:dbl)
    n132 = shared-variable ".\\sensorsSharedVars.lvlib\\sonarLeftRaw(V)"(w157) -> ()  [unwired: 1 in, 1 out]
    n133 = Boolean To (0,1)(Boolean=w155) -> (0, 1=w146:i16)
    n134 = Boolean To (0,1)(Boolean=w154) -> (0, 1=w145:i16)
    n135 = Boolean To (0,1)(Boolean=w153) -> (0, 1=w144:i16)
    n136 = Boolean To (0,1)(Boolean=w152) -> (0, 1=w143:i16)
    n137 = Boolean To (0,1)(Boolean=w151) -> (0, 1=w142:i16)
    n138 = Boolean To (0,1)(Boolean=w150) -> (0, 1=w141:i16)
    n139 = Boolean To (0,1)(Boolean=w149) -> (0, 1=w140:i16)
    n140 = Boolean To (0,1)(Boolean=w148) -> (0, 1=w139:i16)
    n141 = Boolean To (0,1)(Boolean=w156) -> (0, 1=w147:i16)
    n142 = disable-structure shown="Disabled" {
      disable-tunnel: w158 -> [w222 _]
      disable-tunnel: w157 -> [w221 _]
      disable-tunnel: w147 -> [w220 _]
      disable-tunnel: w146 -> [w219 _]
      disable-tunnel: w145 -> [w218 _]
      disable-tunnel: w144 -> [w217 _]
      disable-tunnel: w143 -> [w216 _]
      disable-tunnel: w142 -> [w215 _]
      disable-tunnel: w141 -> [w214 _]
      disable-tunnel: w140 -> [w213 _]
      disable-tunnel: w139 -> [w212 _]
      frame Disabled {
        w196 = "Robot_Data" ("Group")
        n143 = shared-variable ".\\TDMS.lvlib\\TDMS DevRef"() -> (w195:T23)  [unwired: 1 in, 1 out]
        n144 = call <userlib>:"Logger_Log_Data.vi"("Data"=w222, "Channel"="Sonar_Left_Inches", "Group"=w196, "TDMS DevRef"=w195) -> ()  [unwired: 7 in, 1 out]
        n145 = call <userlib>:"Logger_Log_Data.vi"("Data"=w221, "Channel"="Sonar_Left_Raw", "Group"=w196, "TDMS DevRef"=w195) -> ()  [unwired: 7 in, 1 out]
        n146 = call <userlib>:"Logger_Log_Data.vi"("Data"=0.0, "Channel"="Sonar_Right_Inches", "Group"=w196, "TDMS DevRef"=w195) -> ()  [unwired: 7 in, 1 out]
        n147 = call <userlib>:"Logger_Log_Data.vi"("Data"=0.0, "Channel"="Sonar_Right_Raw", "Group"=w196, "TDMS DevRef"=w195) -> ()  [unwired: 7 in, 1 out]
        n148 = call <userlib>:"Logger_Log_Data.vi"("Data"=w220, "Channel"="Hatch_Panel_IR_Detect", "Group"=w196, "TDMS DevRef"=w195) -> ()  [unwired: 7 in, 1 out]
        n149 = call <userlib>:"Logger_Log_Data.vi"("Data"=w219, "Channel"="Climb_IR_Powered_Right", "Group"=w196, "TDMS DevRef"=w195) -> ()  [unwired: 7 in, 1 out]
        n150 = call <userlib>:"Logger_Log_Data.vi"("Data"=w218, "Channel"="Climb_IR_Powered_Left", "Group"=w196, "TDMS DevRef"=w195) -> ()  [unwired: 7 in, 1 out]
        n151 = call <userlib>:"Logger_Log_Data.vi"("Data"=w217, "Channel"="Climb_IR_Skid_Left", "Group"=w196, "TDMS DevRef"=w195) -> ()  [unwired: 7 in, 1 out]
        n152 = call <userlib>:"Logger_Log_Data.vi"("Data"=w216, "Channel"="Climb_IR_Skid_Right", "Group"=w196, "TDMS DevRef"=w195) -> ()  [unwired: 7 in, 1 out]
        n153 = call <userlib>:"Logger_Log_Data.vi"("Data"=w215, "Channel"="Line_IR_Front_Left", "Group"=w196, "TDMS DevRef"=w195) -> ()  [unwired: 7 in, 1 out]
        n154 = call <userlib>:"Logger_Log_Data.vi"("Data"=w214, "Channel"="Line_IR_Front_Right", "Group"=w196, "TDMS DevRef"=w195) -> ()  [unwired: 7 in, 1 out]
        n155 = call <userlib>:"Logger_Log_Data.vi"("Data"=w213, "Channel"="Line_IR_Rear_Left", "Group"=w196, "TDMS DevRef"=w195) -> ()  [unwired: 7 in, 1 out]
        n156 = call <userlib>:"Logger_Log_Data.vi"("Data"=w212, "Channel"="Line_IR_Rear_Right", "Group"=w196, "TDMS DevRef"=w195) -> ()  [unwired: 7 in, 1 out]
      }
      frame Enabled {
      }
    }
    n157 = disable-structure shown="Disabled" {
      disable-tunnel: w177 -> [w237 _]
      disable-tunnel: w176 -> [w236 _]
      frame Disabled {
        w232 = "Robot_Data" ("Group")
        n158 = shared-variable ".\\TDMS.lvlib\\TDMS DevRef"() -> (w231:T23)  [unwired: 1 in, 1 out]
        n159 = Boolean To (0,1)(Boolean=w236) -> (0, 1=w234:i16)
        n160 = call <userlib>:"Logger_Log_Data.vi"("Data"=w234, "Channel"="Sensor_Loop_Late", "Group"=w232, "TDMS DevRef"=w231) -> ()  [unwired: 7 in, 1 out]
        n161 = call <userlib>:"Logger_Log_Data.vi"("Data"=w237, "Channel"="Sensor_Loop_Duration", "Group"=w232, "TDMS DevRef"=w231) -> ()  [unwired: 7 in, 1 out]
      }
      frame Enabled {
      }
    }
    n162 = shared-variable ".\\sensorsSharedVars.lvlib\\yawWind"(w174) -> ()  [unwired: 1 in, 1 out]
    n163 = shared-variable ".\\sensorsSharedVars.lvlib\\pitchWind"(w173) -> ()  [unwired: 1 in, 1 out]
    n164 = shared-variable ".\\sensorsSharedVars.lvlib\\rollwind"(w172) -> ()  [unwired: 1 in, 1 out]
    n165 = disable-structure shown="Disabled" {
      disable-tunnel: w174 -> [w230 _]
      disable-tunnel: w173 -> [w229 _]
      disable-tunnel: w172 -> [w228 _]
      frame Disabled {
        w223 = "Robot_Data" ("Group")
        n166 = shared-variable ".\\TDMS.lvlib\\TDMS DevRef"() -> (w224:T23)  [unwired: 1 in, 1 out]
        n167 = call <userlib>:"Logger_Log_Data.vi"("Data"=w230, "Channel"="IMU_Yaw", "Group"=w223, "TDMS DevRef"=w224) -> ()  [unwired: 7 in, 1 out]
        n168 = call <userlib>:"Logger_Log_Data.vi"("Data"=w229, "Channel"="IMU_Roll", "Group"=w223, "TDMS DevRef"=w224) -> ()  [unwired: 7 in, 1 out]
        n169 = call <userlib>:"Logger_Log_Data.vi"("Data"=w228, "Channel"="IMU_Pitch", "Group"=w223, "TDMS DevRef"=w224) -> ()  [unwired: 7 in, 1 out]
      }
      frame Enabled {
      }
    }
    n170 = case shown="False" w175 {
      frame False {
      }
      frame True {
        n171 = call "sensorTestOutput.vi"() -> ()  [unwired: 12 in]
      }
    }
    n172 = shared-variable ".\\ControlRoom.lvlib\\SensorsPeriod"() -> (w178:i64)  [unwired: 1 in, 1 out]
    n173 = disable-structure shown="Disabled" {
      disable-tunnel: w178 -> [w194 _]
      frame Disabled {
        n174 = shared-variable ".\\TDMS.lvlib\\TDMS DevRef"() -> (w192:T23)  [unwired: 1 in, 1 out]
        n175 = call <userlib>:"Logger_Log_Data.vi"("Data"=w194, "Channel"="Sensor_Loop_Period", "Group"="Robot_Data", "TDMS DevRef"=w192) -> ()  [unwired: 7 in, 1 out]
      }
      frame Enabled {
      }
    }
    n176 = node-c288(w178) -> ()  [unwired: 1 out]
  }
  n177 = node-c288(w15) -> ()  [unwired: 1 out]
  n178 = node-c288(w40) -> ()  [unwired: 2 out]
